vi "Move to Position.vi"(6 "Speed":dbl, 9 "Z-Position":dbl, 10 "Y-Position":dbl, 11 "X-Position":dbl) -> (3 "G-Code String":string)   [LabVIEW 2017]
doc: "Generates G-Code command to move uArm to a desired XYZ position. \n\n<B>Outputs</B>:\n- X-Position: X-Position to move to.\n- Y-Position: Y-Position to move to.\n- Z-Position: Z-Position to move to. \n- Speed: Speed at which uArm will move to position at. \n\n<B>Outputs</B>: \n- G-Code string: G-Code string to move uArm to specified XYZ position."
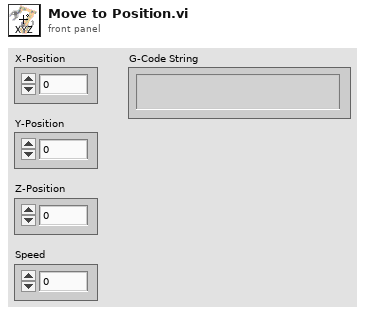
[diagram p1: front panel]
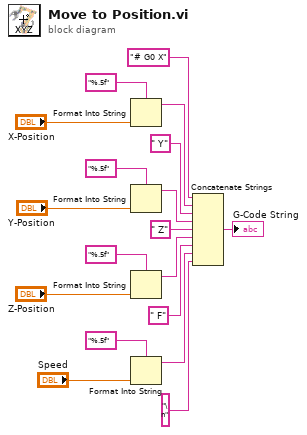
[diagram p0: block diagram]
diagram:
  n1 = Format Into String(format string="%.5f", "X-Position") -> (resulting string=w8:string)  [unwired: 2 in, 1 out]
  n2 = Format Into String(format string="%.5f", "Y-Position") -> (resulting string=w10:string)  [unwired: 2 in, 1 out]
  n3 = Format Into String(format string="%.5f", "Z-Position") -> (resulting string=w5:string)  [unwired: 2 in, 1 out]
  n4 = Format Into String(format string="%.5f", "Speed") -> (resulting string=w1:string)  [unwired: 2 in, 1 out]
  n5 = Concatenate Strings("# G0 X" ("string"), w8, " Y" ("string"), w10, " Z" ("string"), w5, " F" ("string"), w1, "\n" ("string")) -> (→"G-Code String":string)
